vi "Query Assert Status.vi"(11 "TestManagerMsg.Assertion in":refnum<class "TestManagerMsg.Assertion.lvclass">) -> (0 "upstream error":errorcluster, 1 "Skipped":bool, 2 "Passed":bool, 3 "TestManagerMsg.Assertion out":refnum<class "TestManagerMsg.Assertion.lvclass">)   [LabVIEW 2013, in "Caraya.lvlib" / "TestManagerMsg.Assertion.lvclass"]
uses:
  TestManagerMsg.Assertion.lvclass
  TestManagerMsg.Assertion.lvclass/TestManagerMsg.Assertion.ctl
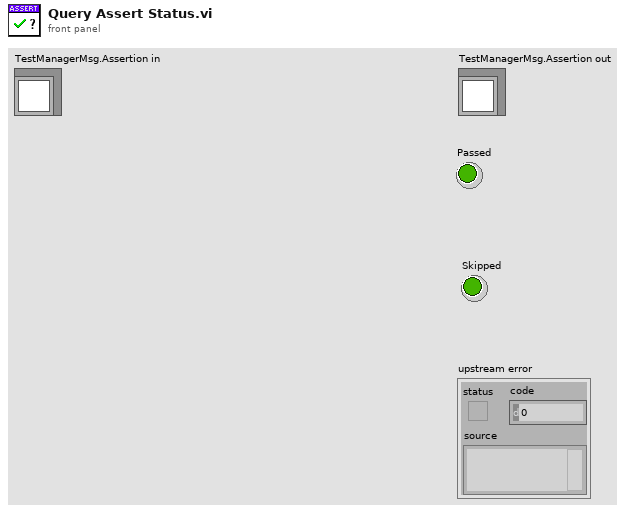
[diagram p1: front panel]
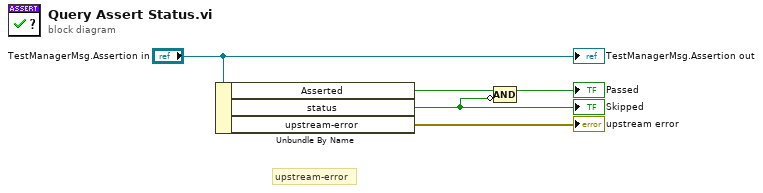
[diagram p0: block diagram]
diagram:
  # "upstream-error"
  n1 = Unbundle By Name("TestManagerMsg.Assertion in") -> ("Asserted"=w4:bool, "status"=w1:bool, "upstream-error"=→"upstream error":errorcluster)
  "Skipped" <- w1
  n2 = Compound Arithmetic op=AND(w4, invert w1) -> (→"Passed":bool)
  "TestManagerMsg.Assertion out" <- "TestManagerMsg.Assertion in"
